vi "GetHeadingLevel.vi"(8 "error in (no error)":errorcluster, 11 "Heading in":refnum<class "Heading.lvclass">) -> (0 "error out":errorcluster, 2 "HeadingLevel":T1(ring), 3 "Heading out":refnum<class "Heading.lvclass">)   [LabVIEW 2021, in "Markdown.lvlib" / "Heading.lvclass"]
uses:
  Heading.lvclass
  Heading.lvclass/Heading.ctl
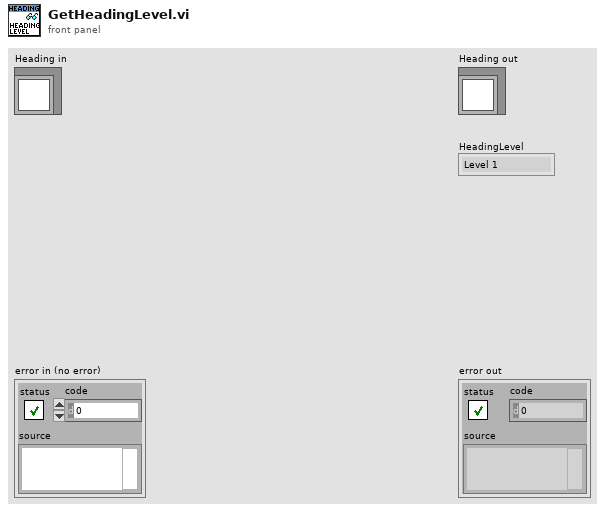
[diagram p1: front panel]
types:
  T1 = enum16{"Level 1", "Level 2", "Level 3", "Level 4", "Level 5", "Level 6"}
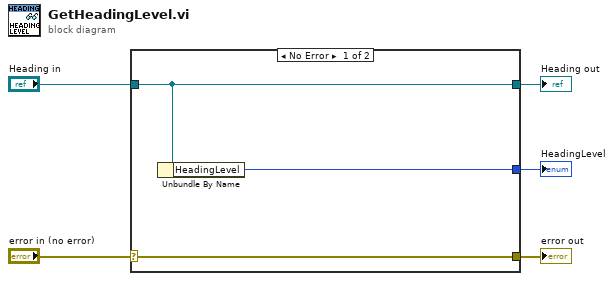
[diagram p0: block diagram]
diagram:
  n1 = case shown="No Error" "error in (no error)" {
    selector: "error in (no error)" -> [w8 w9]
    tunnel: [w8 w9] -> w4
    tunnel: [w7 w10] -> w2
    tunnel: "Heading in" -> [w7 w10]
    tunnel: [w6 _] -> w1
    frame No Error {
      n2 = Unbundle By Name(w7) -> ("HeadingLevel"=w6:T1)
    }
    frame Error {
    }
  }
  "error out" <- w4
  "Heading out" <- w2
  "HeadingLevel" <- w1
